vi "CloseConnection.vi"(8 "error in (no error)":errorcluster, 10 "Connection number":i32, 11 "TCP_ClientWindow_Controller in":refnum<class "TCP_ClientWindow_Controller.lvclass">) -> (0 "error out":errorcluster, 3 "TCP_ClientWindow_Controller out":refnum<class "TCP_ClientWindow_Controller.lvclass">)   [LabVIEW 2023, in "TCP_Client_Window.lvlib" / "TCP_ClientWindow_Controller.lvclass"]
uses:
  TCP_ClientWindow_Controller.lvclass
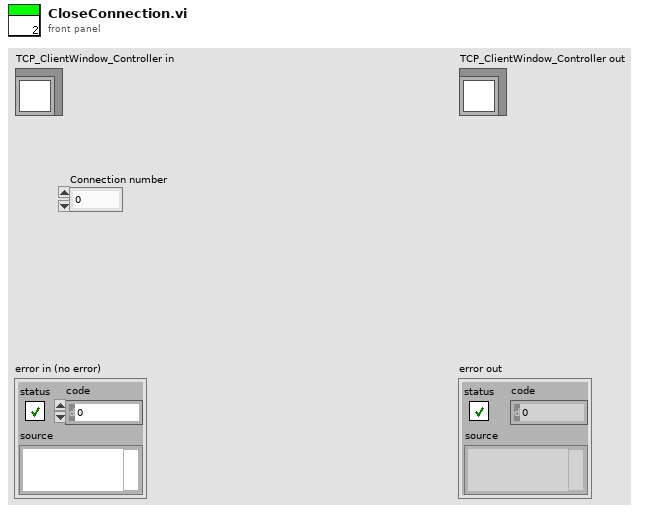
[diagram p1: front panel]
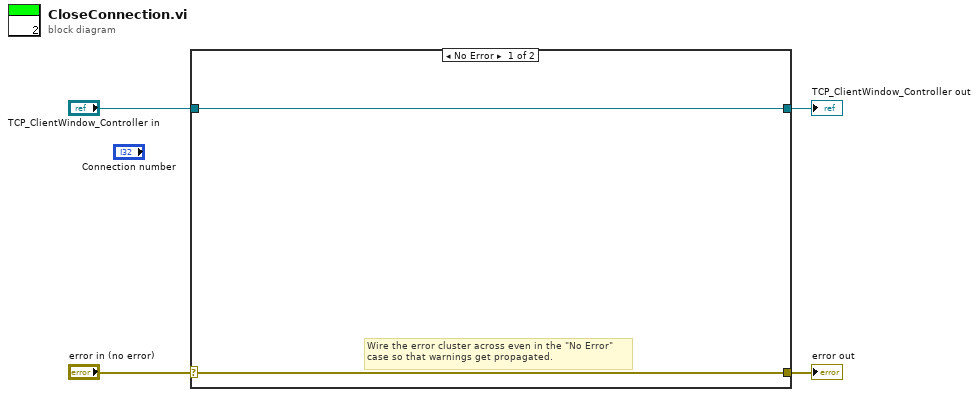
[diagram p0: block diagram]
diagram:
  n1 = case shown="No Error" "error in (no error)" {
    selector: "error in (no error)" -> [w5 w8]
    tunnel: [w5 w8] -> w3
    tunnel: [w6 w7] -> w1
    tunnel: "TCP_ClientWindow_Controller in" -> [w6 w7]
    frame No Error {
      # "Wire the error cluster across even in the \"No Error\"\ncase so that warnings get propagated."
    }
    frame Error {
    }
  }
  "error out" <- w3
  "TCP_ClientWindow_Controller out" <- w1
